vi "init.vi"(8 "error in":errorcluster, 11 "MBParam in":refnum<class "Param.lvclass">) -> (0 "error":errorcluster, 3 "MBParam out":refnum<class "Param.lvclass">)   [LabVIEW 2021, in "Param.lvlib" / "Param.lvclass"]
uses:
  Param.lvclass
  Param.lvclass/Param.ctl
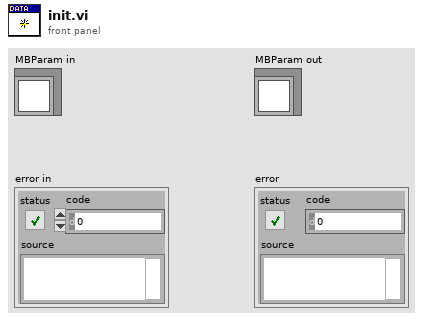
[diagram p1: front panel]
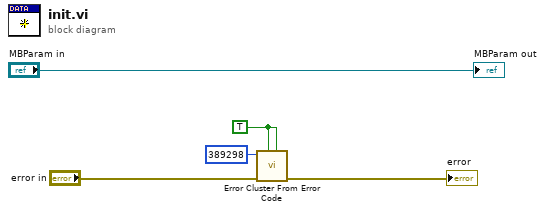
[diagram p0: block diagram]
diagram:
  w1 = TRUE ("show call chain? (False)")
  n1 = call <vilib>:"Error Cluster From Error Code.vi"("is warning? (False)"=w1, "show call chain? (False)"=w1, "error in (no error)"="error in", "error code (0)"=389298) -> ("error out"=→"error":errorcluster)  [unwired: 5 in]
  "MBParam out" <- "MBParam in"
